vi "Wheel PID SetPoint.vi"(2 "Wheel  PID SetPoint Input Array":dbl[](array[numeric])) -> (0 "Wheel  PID SetPoint output Array":dbl[](array[numeric]))   [LabVIEW 2015]
panel:
  in  "Omega":dbl
  out "v right wheel":dbl
  out "v left wheel":dbl
  out "Left Side Setpoint":dbl
  out "Right Side Setpoint":dbl
  in  "Wheel Radius":dbl=0.25 format="%#_13g"
  in  "Track Width":dbl=2.5 format="%#_13g"
  in  "Desired Velocity":dbl
  out "max v":dbl
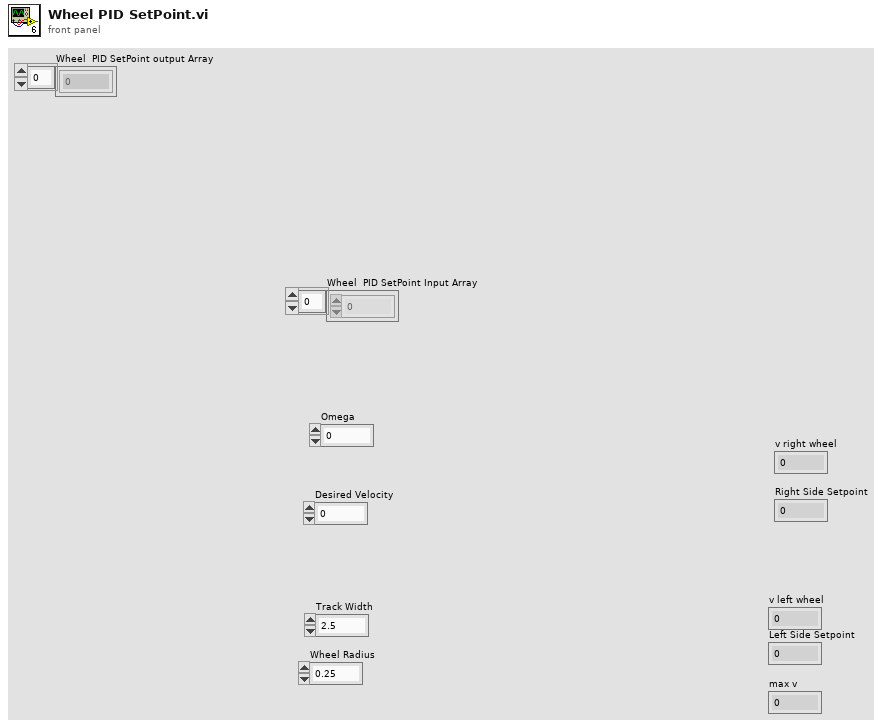
[diagram p1: front panel]
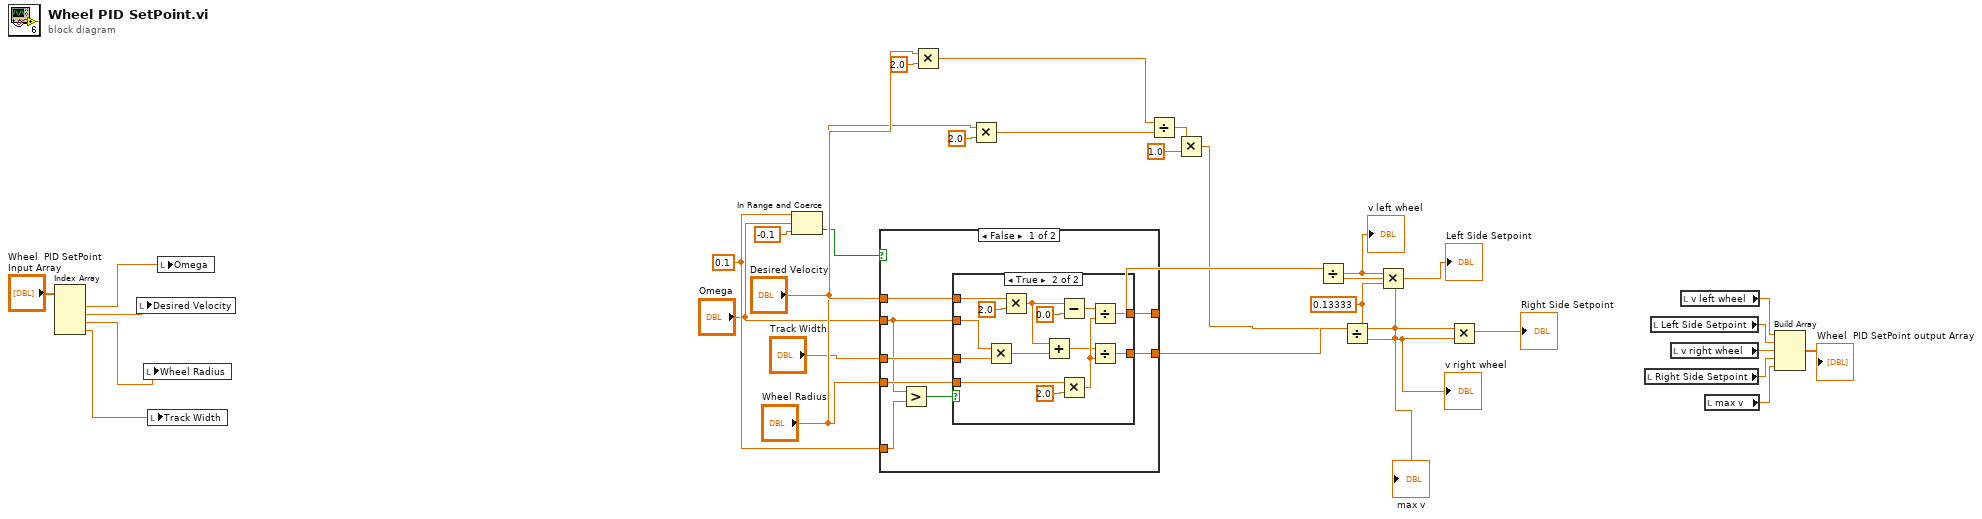
[diagram p0: block diagram]
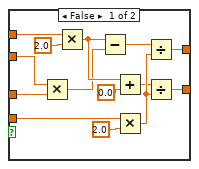
[diagram p2: hidden frame]
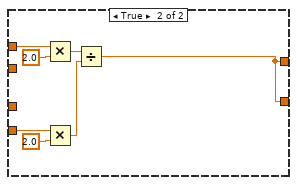
[diagram p3: hidden frame]
diagram:
  w17 = 0.13333 ("y")
  w32 = 0.1 ("upper limit")
  n1 = Index Array(array="Wheel  PID SetPoint Input Array") -> (element #1=w11:dbl, element #2=w10:dbl, element #3=w9:dbl, element #4=w8:dbl)  [unwired: 4 in]
  n2 = local write "Desired Velocity"(w10) -> ()
  n3 = local write "Wheel Radius"(w9) -> ()
  n4 = local write "Track Width"(w8) -> ()
  n5 = local write "Omega"(w11) -> ()
  n6 = In Range and Coerce(upper limit=w32, x="Omega", lower limit=-0.1) -> (In Range?=w21:bool)  [unwired: 1 out]
  n7 = case shown="False" w21 {
    tunnel: [w40 w71] -> w20
    tunnel: [w39 w71] -> w19
    tunnel: "Omega" -> [w35 _]
    tunnel: "Wheel Radius" -> [w37 w70]
    tunnel: "Track Width" -> [w36 _]
    tunnel: "Desired Velocity" -> [w38 w69]
    tunnel: w32 -> [w34 _]
    frame False {
      n8 = Greater?(x=w35, y=w34) -> (0:w33:bool)
      n9 = case shown="True" w33 {
        tunnel: [w48 w62] -> w40
        tunnel: [w47 w61] -> w39
        tunnel: w38 -> [w44 w58]
        tunnel: w37 -> [w41 w57]
        tunnel: w35 -> [w43 w56]
        tunnel: w36 -> [w42 w55]
        frame False {
          n10 = Multiply(x=w43, y=w42) -> (x*y=w46:dbl)
          n11 = Multiply(x=w44, y=2.0) -> (x*y=w51:dbl)
          n12 = Subtract(x=w51, y=w46) -> (x-y=w53:dbl)
          n13 = Add(x=w51, y=0.0) -> (x+y=w52:dbl)
          n14 = Multiply(x=w41, y=2.0) -> (x*y=w54:dbl)
          n15 = Divide(x=w53, y=w54) -> (x/y=w48:dbl)
          n16 = Divide(x=w52, y=w54) -> (x/y=w47:dbl)
        }
        frame True {
          n17 = Multiply(x=w56, y=w55) -> (x*y=w60:dbl)
          n18 = Multiply(x=w58, y=2.0) -> (x*y=w65:dbl)
          n19 = Add(x=w65, y=w60) -> (x+y=w66:dbl)
          n20 = Subtract(x=w65, y=0.0) -> (x-y=w67:dbl)
          n21 = Multiply(x=w57, y=2.0) -> (x*y=w68:dbl)
          n22 = Divide(x=w67, y=w68) -> (x/y=w62:dbl)
          n23 = Divide(x=w66, y=w68) -> (x/y=w61:dbl)
        }
      }
    }
    frame True {
      n24 = Multiply(x=w69, y=2.0) -> (x*y=w72:dbl)
      n25 = Multiply(x=w70, y=2.0) -> (x*y=w75:dbl)
      n26 = Divide(x=w72, y=w75) -> (x/y=w71:dbl)
    }
  }
  n27 = Multiply(x="Desired Velocity", y=2.0) -> (x*y=w25:dbl)
  n28 = Multiply(x="Wheel Radius", y=2.0) -> (x*y=w28:dbl)
  n29 = Divide(x=w25, y=w28) -> (x/y=w29:dbl)
  n30 = Multiply(x=w29, y=1.0) -> (x*y=w13:dbl)
  "max v" <- w13
  n31 = Divide(x=w20, y=w13) -> (x/y=w18:dbl)
  "v left wheel" <- w18
  n32 = Divide(x=w19, y=w13) -> (x/y=w16:dbl)
  "v right wheel" <- w16
  n33 = Multiply(x=w18, y=w17) -> (x*y=→"Left Side Setpoint":dbl)
  n34 = Multiply(x=w17, y=w16) -> (x*y=→"Right Side Setpoint":dbl)
  n35 = local read "Right Side Setpoint"() -> (w2:dbl)
  n36 = local read "Left Side Setpoint"() -> (w4:dbl)
  n37 = local read "v right wheel"() -> (w3:dbl)
  n38 = local read "v left wheel"() -> (w5:dbl)
  n39 = local read "max v"() -> (w1:dbl)
  n40 = Build Array(w5, w4, w3, w2, w1) -> (→"Wheel  PID SetPoint output Array":dbl[])
